vi "TestVI_Analyzer.vi"(8 "error in (no error)":errorcluster, 11 "TestCase in":refnum<class "Test Status Updater.lvclass">) -> (0 "error out":errorcluster, 3 "TestCase out":refnum<class "Test Status Updater.lvclass">)   [LabVIEW 2014, in "Test Status Updater.lvclass"]
uses:
  Test Status Updater.lvclass
  <vilib>/addons/_JKI Toolkits/VI Tester/TestCase.llb/TestCase.lvclass
  Core/LabVIEW CI Service/Extensions/VI Analyzer/VI Analyzer/VI Analyzer.lvclass
  Core/LabVIEW CI Service/Extensions/VI Analyzer/VI Analyzer/VI Analyzer - STYP.ctl
  Core/LabVIEW CI Service/Classes/Status Updater/Status Updater.lvclass
  Core/LabVIEW CI Service/Classes/Job/Job.lvclass
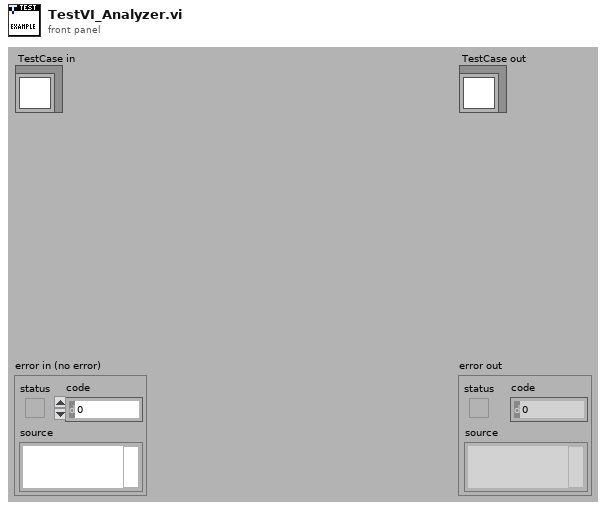
[diagram p1: front panel]
types:
  T1 = typedef "VI Analyzer - STYP.ctl" = cluster{"Executor_Number":string, "Workspace_Path":string, "Test File":string}
  T2 = cluster{"Event Registration Refnum":refnum<event-registration>, "Event Registration Refnum":refnum<event-registration>}
  T3 = typedef "Job Results - STYP.ctl" = cluster{"Status":u16, "Text":string, "Executor Number":i32}
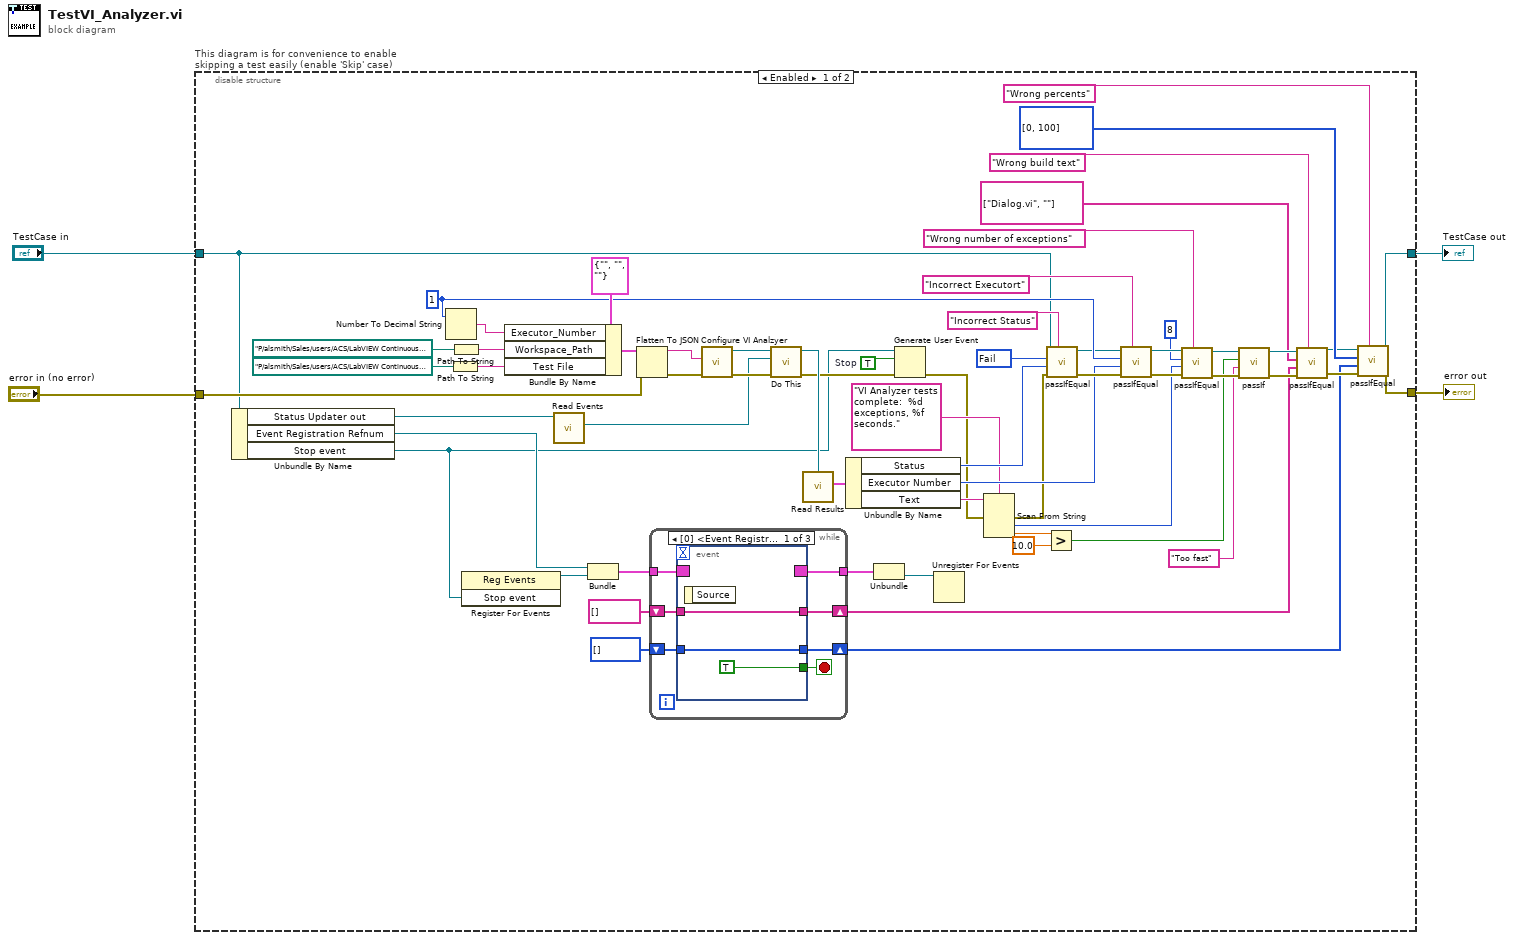
[diagram p0: block diagram]
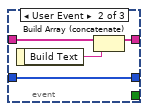
[diagram p2: hidden frame]
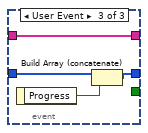
[diagram p3: hidden frame]
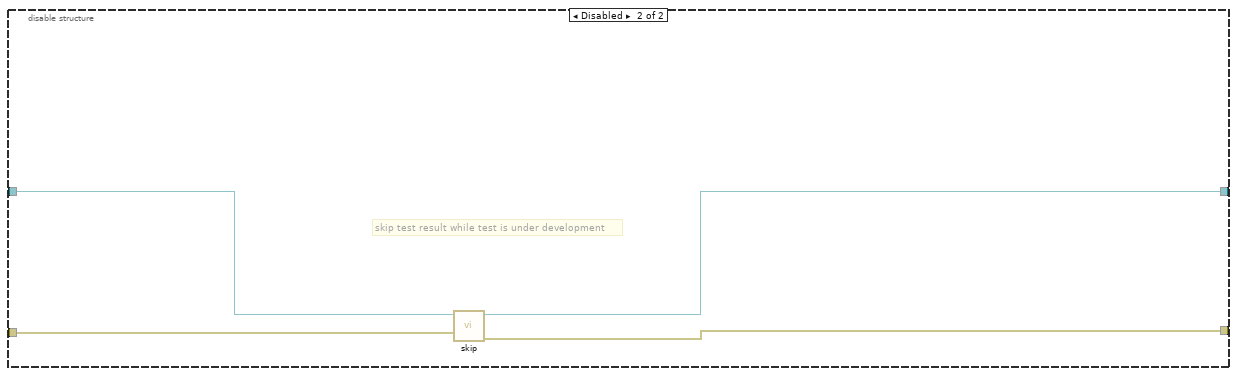
[diagram p4: hidden frame]
diagram:
  n1 = disable-structure "This diagram is for convenience to enable skipping a test easily (enable 'Skip' case)" shown="Enabled" {
    disable-tunnel: "TestCase in" -> [w14 w88]
    disable-tunnel: [w66 w86] -> w1
    disable-tunnel: [w65 w87] -> w3
    disable-tunnel: "error in (no error)" -> [w45 w85]
    frame Enabled {
      w10 = TRUE  # Stop
      w42 = u16 500 items=["Service Error"=504, "Abort"=503, "Fail"=500, "Pass"=200] ("Status")
      w40 = 1 ("number")
      n2 = Unbundle By Name(w14) -> ("Status Updater out"=w53:refnum<class "Status Updater.lvclass">, "Event Registration Refnum"=w47:refnum<event-registration>, "Stop event"=w7:refnum<user-event>)
      n3 = Number To Decimal String(number=w40) -> (decimal integer string=w59:string)  [unwired: 1 in]
      n4 = Path To String(path=path "P:/alsmith/Sales/users/ACS/LabVIEW Continuous Integration/Jenkins Sample Project/Jenkins Sample Project.cfg" ("Test File")) -> (string=w58:string)
      n5 = Path To String(path=path "P:/alsmith/Sales/users/ACS/LabVIEW Continuous Integration/Test/VI Analyzer Job Test Code" ("Workspace Path")) -> (string=w62:string)
      n6 = register-events(w7) -> (reference out=w50:refnum<event-registration>)  [unwired: 2 in, 1 out]
      n7 = Bundle By Name(cluster=T1 {"Executor_Number"="", "Workspace_Path"="", "Test File"=""} ("VI Analyzer - STYP.ctl"), "Executor_Number"=w59, "Workspace_Path"=w62, "Test File"=w58) -> (w56:T1)
      n8 = call "Read Events.vi"("Status Updater in"=w53) -> ("Status Events"=w52:refnum<class "Status Events.lvclass">)  [unwired: 10 in]
      n9 = Bundle("Event Registration Refnum"=w47, "Event Registration Refnum"=w50) -> (w51:T2)  [unwired: 1 in]
      n10 = Flatten To JSON(anything=w56, error in (no error)=w45) -> (JSON string=w60:string, 11:w61:errorcluster)  [unwired: 1 in]
      n11 = while {
        tunnel: w51 -> [w73]
        shift-right: [w70] -> w18
        shift-left: string[] [] -> [w71]
        shift-right: [w68] -> w11
        shift-left: u32[] [] -> [w69]
        tunnel: [w67] -> w6
        stop <- w72 stop-if-true
        n12 = event shown="[0] <Event Registration Refnum.Stop event>: User Event" {
          selector: w73 -> [_ _ _]
          dyn-events: [_ _ _] -> w67
          timeout: _ -> [_ _ _]
          tunnel: [TRUE _ _] -> w72
          tunnel: w71 -> [w75 w80 w84]
          tunnel: [w75 w79 w84] -> w70
          tunnel: w69 -> [w74 w77 w83]
          tunnel: [w74 w77 w81] -> w68
          event User Event {
            n13 = event-data() -> ()  [unwired: 1 in, 1 out]
          }
          event User Event {
            n14 = event-data() -> ("Build Text"=w78:string)  [unwired: 1 in]
            n15 = Build Array (concatenate)(w80, w78) -> (w79:string[])
          }
          event User Event {
            n16 = event-data() -> ("Progress"=w82:u32)  [unwired: 1 in]
            n17 = Build Array (concatenate)(w83, w82) -> (w81:u32[])
          }
        }
      }
      n18 = call "Configure VI Analzyer.vi"("error in (no error)"=w61, "JSON String"=w60) -> ("error out"=w64:errorcluster, "VI Analyzer out"=w63:refnum<class "VI Analyzer.lvclass">)  [unwired: 8 in]
      n19 = call-dynamic "Do This.vi"("error in (no error)"=w64, "Status Events"=w52, "VI Analyzer in"=w63) -> ("error out"=w9:errorcluster, "VI Analyzer out"=w46:refnum<class "VI Analyzer.lvclass">)  [unwired: 7 in]
      n20 = call "Read Results.vi"("Job in"=w46) -> ("Results"=w44:T3)  [unwired: 10 in]
      n21 = Unbundle By Name(w44) -> ("Status"=w43:u16, "Executor Number"=w39:i32, "Text"=w38:string)
      n22 = Unbundle(w6) -> ("Event Registration Refnum"=w5:refnum<event-registration>)  [unwired: 1 out]
      n23 = Generate User Event(user event=w7, event data cluster=w10, error in=w9) -> (error out=w8:errorcluster)  [unwired: 1 in, 1 out]
      n24 = Unregister For Events(event registration refnum=w5) -> ()  [unwired: 1 in, 1 out]
      n25 = Scan From String(format string="VI Analyzer tests complete:  %d exceptions, %f seconds." ("Text"), input string=w38, error in=w8) -> (error out=w36:errorcluster, output 1=w32:i32, output 2=w28:dbl)  [unwired: 3 in, 2 out]
      n26 = Greater?(x=w28, y=10.0) -> (0:w26:bool)
      n27 = call-dynamic "passIfEqual.vi"(7:"Incorrect Status" ("custom report message (\"\")"), "error in (no error)"=w36, "y"=w43, "x"=w42, "TestCase in"=w14) -> ("error out"=w41:errorcluster, "TestCase out"=w34:refnum<class "Test Status Updater.lvclass">)  [unwired: 5 in]
      n28 = call-dynamic "passIfEqual.vi"(7:"Incorrect Executort" ("custom report message (\"\")"), "error in (no error)"=w41, "y"=w39, "x"=w40, "TestCase in"=w34) -> ("error out"=w35:errorcluster, "TestCase out"=w33:refnum<class "Test Status Updater.lvclass">)  [unwired: 5 in]
      n29 = call-dynamic "passIfEqual.vi"(7:"Wrong number of exceptions" ("custom report message (\"\")"), "error in (no error)"=w35, "y"=w32, "x"=8, "TestCase in"=w33) -> ("error out"=w30:errorcluster, "TestCase out"=w29:refnum<class "Test Status Updater.lvclass">)  [unwired: 5 in]
      n30 = call-dynamic "passIf.vi"("error in (no error)"=w30, "message (\"\")"="Too fast" ("message (\"\")"), "pass"=w26, "TestCase in"=w29) -> ("error out"=w20:errorcluster, "TestCase out"=w19:refnum<class "Test Status Updater.lvclass">)  [unwired: 6 in]
      n31 = call-dynamic "passIfEqual.vi"(7:"Wrong build text" ("custom report message (\"\")"), "error in (no error)"=w20, "y"=w18, "x"=string[] ["Dialog.vi", ""] ("Steps"), "TestCase in"=w19) -> ("error out"=w21:errorcluster, "TestCase out"=w13:refnum<class "Test Status Updater.lvclass">)  [unwired: 5 in]
      n32 = call-dynamic "passIfEqual.vi"(7:"Wrong percents" ("custom report message (\"\")"), "error in (no error)"=w21, "y"=w11, "x"=u32[] [0, 100] ("Progress Percents"), "TestCase in"=w13) -> ("error out"=w65:errorcluster, "TestCase out"=w66:refnum<class "Test Status Updater.lvclass">)  [unwired: 5 in]
    }
    frame Disabled {
      # "skip test result while test is under development"
      n33 = call <vilib>:"skip.vi"("error in (no error)"=w85, "TestCase in"=w88) -> ("error out"=w87:errorcluster, "TestCase out"=w86:refnum<class "Test Status Updater.lvclass">)  [unwired: 8 in]
    }
  }
  "error out" <- w3
  "TestCase out" <- w1
